vi "parse-sce-pannel-list.vi"(11 "sce-pannel-list":T1(array[cluster]) {"pannel"."ID" format="%02x"}) -> (2 "sce-regulate-list":T1(array[cluster]), 3 "sce-pannel-list out":T2(array[cluster]) {"pannel"."ID" format="%02x"})   [LabVIEW 2019]
panel:
  out "数组":T1(array[cluster])
  in  "sce-pannel-list 3":T1(array[cluster])
  in  "sce-pannel-list 2":T1(array[cluster])
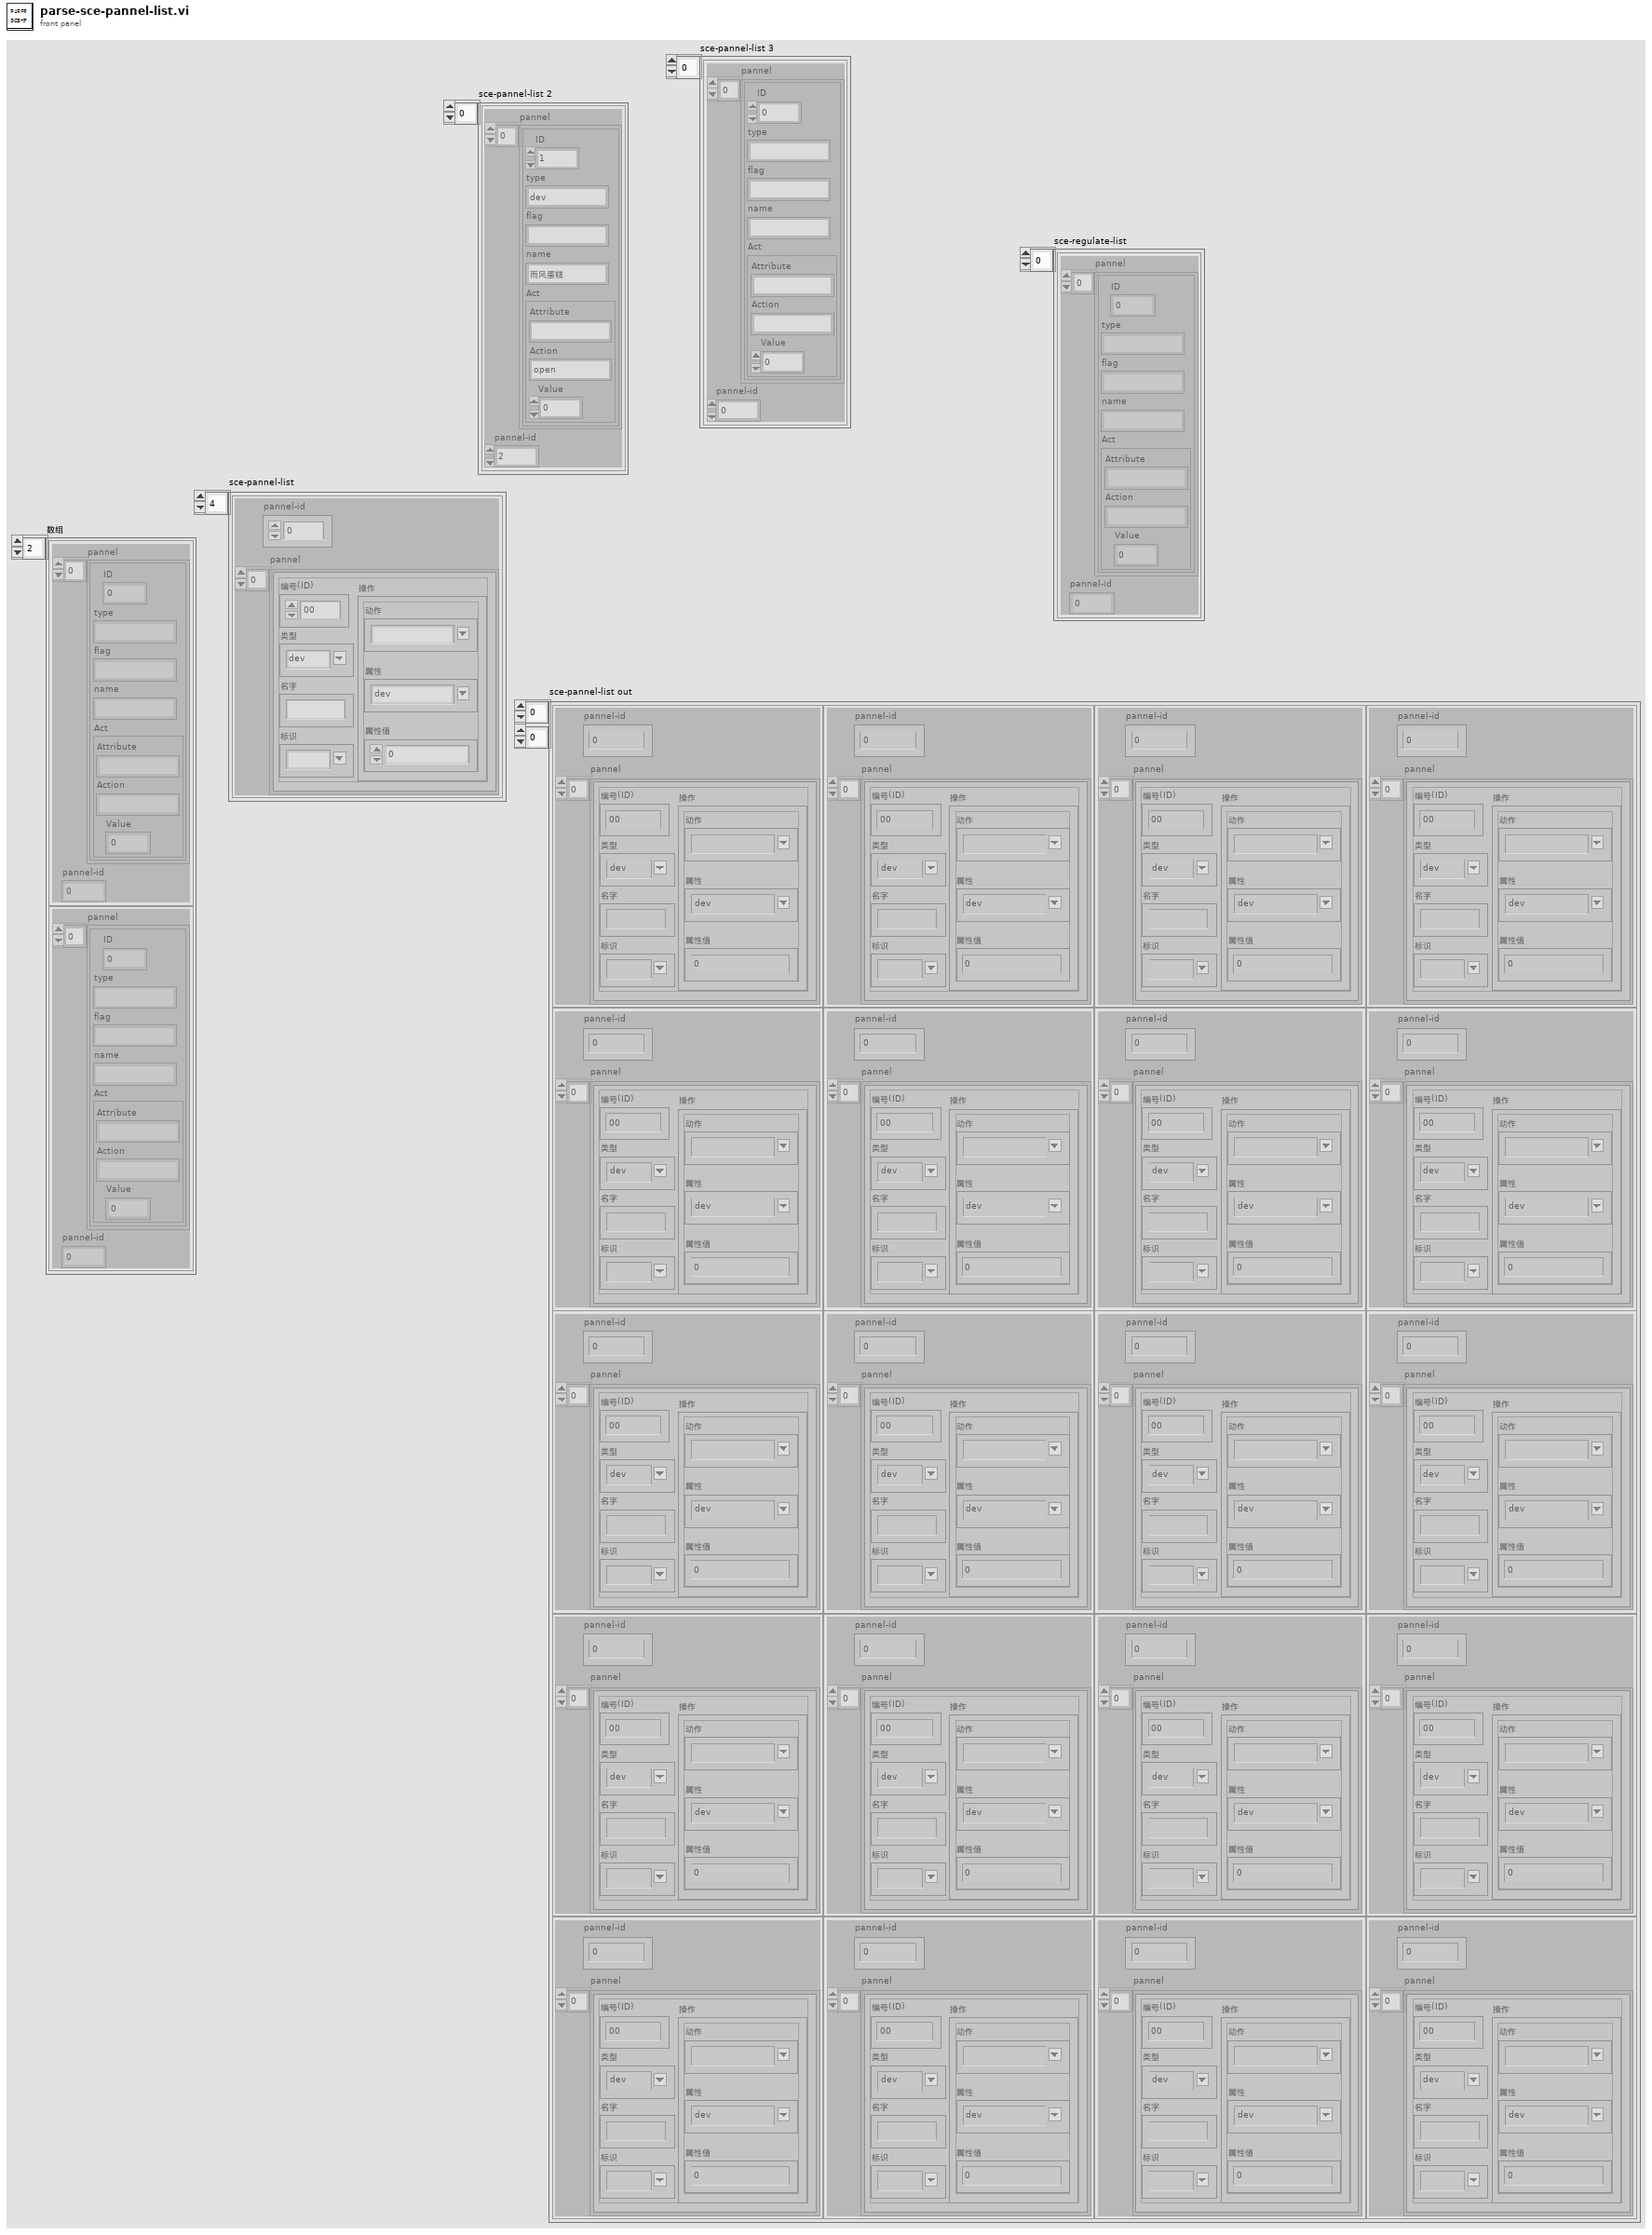
[diagram p1: front panel]
types:
  T1 = cluster{"pannel":cluster{"ID":u8, "type":string, "flag":string, "name":string, "Act":cluster{"Attribute":string, "Action":string, "Value":dbl}}[], "pannel-id":dbl}[]
  T2 = cluster{"pannel":cluster{"ID":u8, "type":string, "flag":string, "name":string, "Act":cluster{"Attribute":string, "Action":string, "Value":dbl}}[], "pannel-id":dbl}[][]
  T3 = cluster{"ID":u8, "type":string, "flag":string, "name":string, "Act":cluster{"Attribute":string, "Action":string, "Value":dbl}}[]
  T4 = cluster{"ID":u8, "type":string, "flag":string, "name":string, "Act":cluster{"Attribute":string, "Action":string, "Value":dbl}}
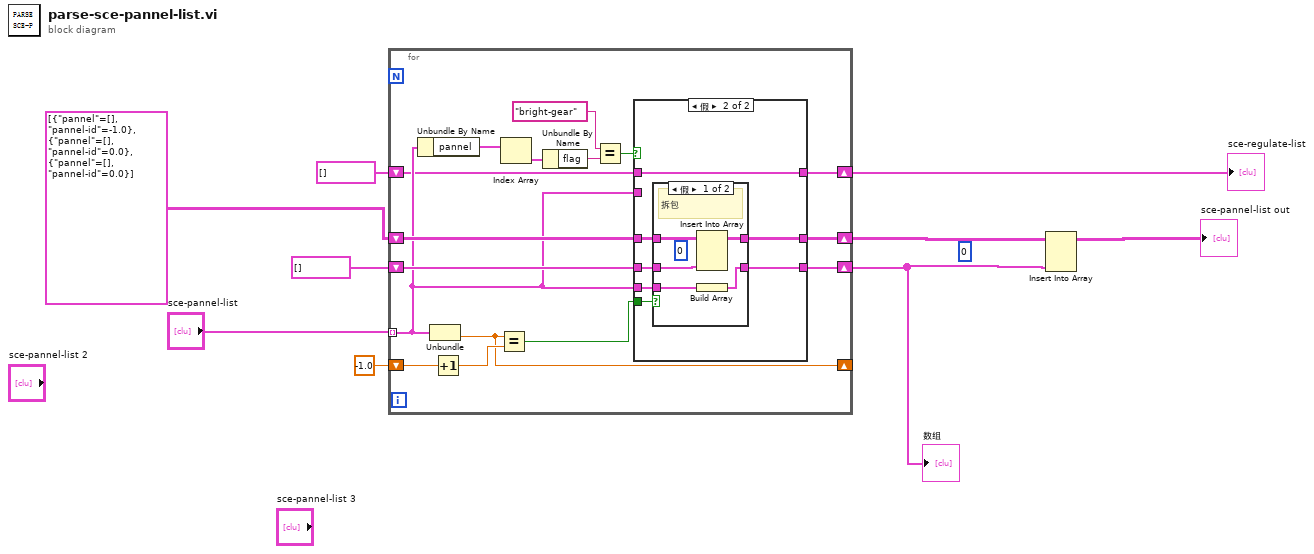
[diagram p0: block diagram]
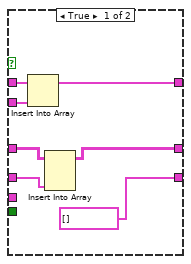
[diagram p2: hidden frame]
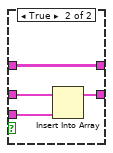
[diagram p3: hidden frame]
diagram:
  (unwired) 0 ("索引 (行)")
  n1 = for {
    tunnel: "sce-pannel-list" -> [w12] mode=indexing
    shift-right: [w22] -> _
    shift-left: -1.0 ("pannel-id") -> [w25]
    shift-right: [w21] -> w2
    shift-left: T1 [] -> [w20]
    shift-right: [w19] -> w6
    shift-left: T2 [[{"pannel"=[], "pannel-id"=-1.0}, {"pannel"=[], "pannel-id"=0.0}, {"pannel"=[], "pannel-id"=0.0}]] ("sce-pannel-list out") -> [w18]
    shift-right: [w11] -> w4
    shift-left: T1 [] -> [w10]
    n2 = Unbundle By Name(w12) -> ("pannel"=w17:T3)
    n3 = Unbundle(w12) -> ("pannel-id"=w22:dbl)  [unwired: 1 out]
    n4 = Increment(x=w25) -> (x+1=w24:dbl)
    n5 = Equal?(x=w22, y=w24) -> (x = y?=w23:bool)
    n6 = Index Array(array=w17) -> (element=w15:T4)  [unwired: 1 in]
    n7 = Unbundle By Name(w15) -> ("flag"=w14:string)
    n8 = Equal?(x="bright-gear", y=w14) -> (x = y?=w13:bool)
    n9 = case shown="假" w13 {
      tunnel: w23 -> [_ w39]
      tunnel: [T1 [] w38] -> w21
      tunnel: w20 -> [w26 w37]
      tunnel: [w27 w36] -> w19
      tunnel: w18 -> [w28 w35]
      tunnel: w12 -> [_ w34]
      tunnel: w12 -> [w31 _]
      tunnel: [w30 w33] -> w11
      tunnel: w10 -> [w32 w33]
      frame True {
        n10 = Insert Into Array(array=w32, new element=w31) -> (w30:T1)  [unwired: 1 in]
        n11 = Insert Into Array(array=w28, new element=w26) -> (w27:T2)  [unwired: 2 in]
      }
      frame False {
        n12 = case shown="假" w39 {
          tunnel: w34 -> [w40 w48]
          tunnel: [w41 w47] -> w38
          tunnel: w37 -> [w44 w46]
          tunnel: [w43 w45] -> w36
          tunnel: w35 -> [w42 w45]
          frame False {
            (unwired) 0 ("索引 (行)")
            # "拆包"
            n13 = Insert Into Array(array=w42, new element=w44) -> (w43:T2)  [unwired: 2 in]
            n14 = Build Array(w40) -> (w41:T1)
          }
          frame True {
            n15 = Insert Into Array(array=w46, new element=w48) -> (w47:T1)  [unwired: 1 in]
          }
        }
      }
    }
  }
  "sce-regulate-list" <- w4
  "数组" <- w2
  n16 = Insert Into Array(array=w6, new element=w2) -> (→"sce-pannel-list out":T2)  [unwired: 2 in]
